vi "Do.vi"(8 "error in (no error)":errorcluster, 10 "Actor in":refnum<class "Actor.lvclass">, 11 "Set Output Line Msg":refnum<class "Set Output Line Msg.lvclass">) -> (0 "error out":errorcluster, 2 "Actor out":refnum<class "Actor.lvclass">)   [LabVIEW 2017, in "BNT_DAQmx.lvlib" / "Set Output Line Msg.lvclass"]
doc: "This VI delivers the message to the actor by calling the appropriate method(s) on the actor."
uses:
  Set Output Line Msg.lvclass
  <vilib>/ActorFramework/Actor/Actor.lvclass
  C:/User/Brand/LVP/Acc/VacuumHeating/Packages/CSPP_Core/Messages/CSPP_PVUpdate Msg/CSPP_PVUpdate Msg.lvclass
  BNT_DAQmx-MCSV/BNT_DAQmx-MCSV.lvclass
  C:/Program Files (x86)/National Instruments/LabVIEW 2017/vi.lib/ActorFramework/Actor/Actor.lvclass
  CSPP_Core/Messages/CSPP_PVUpdate Msg/CSPP_PVUpdate Msg.lvclass/CSPP_PVUpdate Msg.ctl
  CSPP_Core/Classes/CSPP_ProcessVariables/ProcessVariable/PV.lvclass/PV.ctl
  Set Output Line Msg.lvclass/Set Output Line Msg.ctl
  CSPP_Core/Classes/CSPP_ProcessVariables/ProcessVariable/PV.lvclass
  <vilib>/regexp/Match Regular Expression.xnode
  CSPP_Core/Messages/CSPP_PVUpdate Msg/CSPP_PVUpdate Msg.lvclass
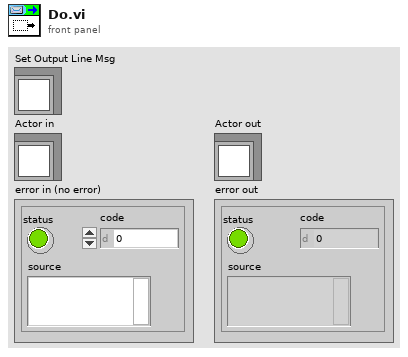
[diagram p1: front panel]
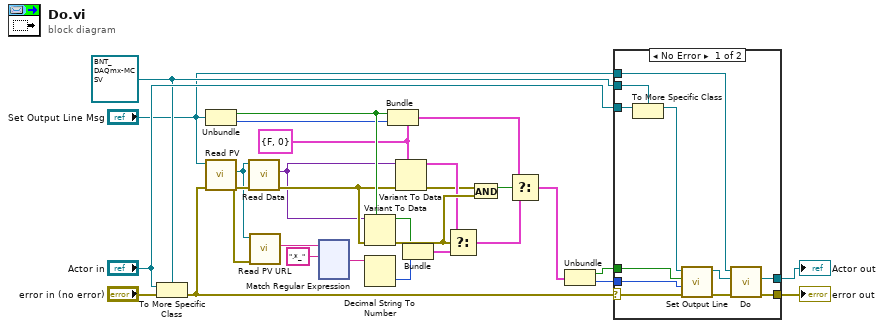
[diagram p0: block diagram]
diagram:
  w6 = cluster{"Enable Channel":bool, "Channel":i32} {"Enable Channel"=FALSE, "Channel"=0} ("Type")
  w25 = refnum<class "BNT_DAQmx-MCSV.lvclass"> refnum ("Actor in")
  n1 = To More Specific Class(target class=w25, reference="Actor in", error in="error in (no error)") -> (error out=w3:errorcluster)  [unwired: 1 out]
  n2 = Unbundle ("Pre-Unbundler")("Set Output Line Msg") -> (w17:bool, w7:i32)
  n3 = call "Read PV.vi"("error in (no error)"=w3, "CS++PVUpdate Msg in"="Set Output Line Msg") -> ("error out"=w14:errorcluster, "PV"=w13:refnum<class "PV.lvclass">)  [unwired: 7 in, 1 out]
  n4 = call "Read Data.vi"("error in (no error)"=w14, "PV in"=w13) -> ("error out"=w16:errorcluster, "Data"=w15:variant)  [unwired: 7 in, 1 out]
  n5 = call "Read PV URL.vi"("error in (no error)"=w14, "PV in"=w13) -> ("PV URL"=w8:string)  [unwired: 7 in, 2 out]
  n6 = xnode "Match Regular Expression"("input string"=w8, "regular expression"=".*_") -> ("after match"=w10:string)  [unwired: 4 in, 4 out]
  n7 = Variant To Data(error in=w16, type=w17, Variant=w15) -> (data=w18:bool, error out=w22:errorcluster)
  n8 = Decimal String To Number(string=w10) -> (number=w11:i32)  [unwired: 2 in, 1 out]
  n9 = Bundle ("Pre-Bundler")(cluster=w6, "Enable Channel"=w17, "Channel"=w7) -> (w5:cluster{"Enable Channel":bool, "Channel":i32})
  n10 = Variant To Data(error in=w16, type=w6, Variant=w15) -> (data=w19:cluster{"Enable Channel":bool, "Channel":i32}, error out=w4:errorcluster)
  n11 = Bundle ("Pre-Bundler")("Value"=w18, w11) -> (w12:cluster{"Value":bool, i32})  [unwired: 1 in]
  n12 = Select ("MainSelect")(t=w19, s=w22, f=w12) -> (s? t:f=w20:cluster{"Value":bool, "Channel":i32})
  n13 = And(x=w4, y=w22) -> (x .and. y?=w21:bool)
  n14 = Select ("MainSelect")(t=w5, s=w21, f=w20) -> (s? t:f=w1:cluster{"Value":bool, "Channel":i32})
  n15 = Unbundle ("Main-Unbundler")(w1) -> ("Value"=w24:bool, "Channel"=w23:i32)
  n16 = case shown="No Error" w3 {
    selector: w3 -> [w40 w42]
    tunnel: [w35 w42] -> w28
    tunnel: [w36 w41] -> w27
    tunnel: "Actor in" -> [w39 w41]
    tunnel: w25 -> [w38 _]
    tunnel: "Set Output Line Msg" -> [w32 _]
    tunnel: w24 -> [w31 _]
    tunnel: w23 -> [w30 _]
    frame No Error {
      n17 = To More Specific Class ("To More Specific Class (internal)")(target class=w38, reference=w39) -> (specific class reference=w37:refnum<class "BNT_DAQmx-MCSV.lvclass">)  [unwired: 1 in, 1 out]
      n18 = call "Set Output Line.vi"("Error In"=w40, "Line"=w30, "Value"=w31, "BNT_DAQmx-MCSV in"=w37) -> ("Error Out"=w34:errorcluster, "BNT_DAQmx-MCSV out"=w33:refnum<class "BNT_DAQmx-MCSV.lvclass">)  [unwired: 6 in]
      n19 = call-parent "Do.vi"("error in (no error)"=w34, "Actor in"=w33, "CS++PVUpdate Msg"=w32) -> ("error out"=w35:errorcluster, "Actor out"=w36:refnum<class "Actor.lvclass">)  [unwired: 7 in]
    }
    frame Error {
    }
  }
  "error out" <- w28
  "Actor out" <- w27
